vi "NI VeriStand - Open Waveform Session.vi"   [LabVIEW 2020, in "NI_VS Custom Device Waveform API.lvlib"]
doc: "Opens a session for reading data from or writing data to a specific waveform or waveforms associated with a custom device. You must manually select the instance to use according to the number of waveforms with which you want to interact, whether the data type of the waveforms is DBL or CDB, and whether you want to read or write waveform data."
uses:
  <vilib>/NI VeriStand/Custom Device Waveform API/NI_VS Custom Device Waveform API.lvlib
  <vilib>/NI VeriStand/Custom Device Waveform API/Multiple Waveforms Write (DBL)/Multiple Waveforms Write (DBL).lvclass
  <vilib>/NI VeriStand/Custom Device Waveform API/Multiple Waveforms Read (DBL)/Multiple Waveforms Read (DBL).lvclass
  <vilib>/NI VeriStand/Custom Device Waveform API/Multiple Waveforms Read (CDB)/Multiple Waveforms Read (CDB).lvclass
  <vilib>/NI VeriStand/Custom Device Waveform API/Multiple Waveforms Write (CDB)/Multiple Waveforms Write (CDB).lvclass
  <vilib>/NI VeriStand/Custom Device Waveform API/Single Waveform Write (CDB)/Single Waveform Write (CDB).lvclass
  <vilib>/NI VeriStand/Custom Device Waveform API/Single Waveform Write (DBL)/Single Waveform Write (DBL).lvclass
  <vilib>/NI VeriStand/Custom Device Waveform API/Single Waveform Read (DBL)/Single Waveform Read (DBL).lvclass
  <vilib>/NI VeriStand/Custom Device Waveform API/Single Waveform Read (CDB)/Single Waveform Read (CDB).lvclass
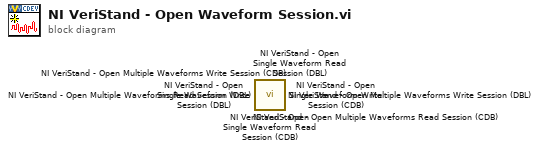
[diagram p0: block diagram]
diagram:
  n1 = call <vilib>:"NI VeriStand - Open Single Waveform Read Session (CDB).vi"() -> ()  [unwired: 10 in, 2 out]
  n2 = call <vilib>:"NI VeriStand - Open Single Waveform Read Session (DBL).vi"() -> ()  [unwired: 10 in, 2 out]
  n3 = call <vilib>:"NI VeriStand - Open Single Waveform Write Session (DBL).vi"() -> ()  [unwired: 10 in, 2 out]
  n4 = call <vilib>:"NI VeriStand - Open Single Waveform Write Session (CDB).vi"() -> ()  [unwired: 10 in, 2 out]
  n5 = call <vilib>:"NI VeriStand - Open Multiple Waveforms Write Session (CDB).vi"() -> ()  [unwired: 10 in, 2 out]
  n6 = call <vilib>:"NI VeriStand - Open Multiple Waveforms Read Session (CDB).vi"() -> ()  [unwired: 10 in, 2 out]
  n7 = call <vilib>:"NI VeriStand - Open Multiple Waveforms Read Session (DBL).vi"() -> ()  [unwired: 10 in, 2 out]
  n8 = call <vilib>:"NI VeriStand - Open Multiple Waveforms Write Session (DBL).vi"() -> ()  [unwired: 10 in, 2 out]
